vi "Periodic Tasks.vi"(8 "error in":errorcluster) -> ()   [LabVIEW 2020]
doc: "This VI runs in parallel to other tasks. It can contain as many user-defined periodic loops as you need. These can carry out PID or other sorts of timed response."
uses:
  <vilib>/Rock Robotics/WPI/Utilities/WPI_GetSetVariantRefNum.vi
  <vilib>/Rock Robotics/WPI/ThirdParty/REV Robotics/REVLib/Typedef/Spark MAX Control Type.ctl
  981LabViewComponents/2022 Robot Global Data.vi
panel:
  out "Sensor Position":dbl
  out "Sensor Velocity":dbl
  out "YRPHfH":T1
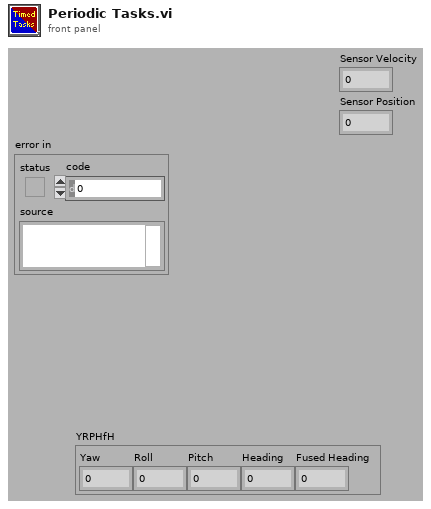
[diagram p1: front panel]
types:
  T1 = cluster{"Yaw":dbl, "Roll":dbl, "Pitch":dbl, "Heading":dbl, "Fused Heading":dbl}
  T2 = typedef "WPI_MotorControlDeviceRef.ctl" = cluster{"DeviceStatus":errorcluster, "Type":T3, "PWM":cluster{"PWM Channel":T4, "DeadBand":T5}, "CAN":cluster{"Device Number":u8, "SetOutput VI Ref":variant, "GetOutput VI Ref":variant, "Enable VI Ref":variant, "Disable VI Ref":variant, "Data":variant}, "Invert":bool, "DIO PWM":cluster{"PWM \"Enable\" Channel":T4, "DIOChannel":T6, "PWM Rate":dbl}}
  T3 = typedef "WPI_MotorControlType.ctl" = enum16{"PWM", "CAN", "DIO PWM"}
  T4 = typedef "FPGA_DIOPWMChannel.ctl" = enum8{"PWM 0", "PWM 1", "PWM 2", "PWM 3", "PWM 4", "PWM 5", "PWM 6", "PWM 7", "PWM 8", "PWM 9", "PWM MXP 0", "PWM MXP 1", "PWM MXP 2", "PWM MXP 3", "PWM MXP 4", "PWM MXP 5", "PWM MXP 6", "PWM MXP 7", "PWM MXP 8", "PWM MXP 9", "Invalid"}
  T5 = typedef "WPI_PWMDeadband.ctl" = cluster{"Name":string, "maxPositivePwm":i32, "minPositivePwm":i32, "centerPwm":i32, "maxNegativePwm":i32, "minNegativePwm":i32, "angularRange":u16}
  T6 = typedef "FPGA_DIOChannel.ctl" = enum8{"DIO 0", "DIO 1", "DIO 2", "DIO 3", "DIO 4", "DIO 5", "DIO 6", "DIO 7", "DIO 8", "DIO 9", "DIO MXP 0", "DIO MXP 1", "DIO MXP 2", "DIO MXP 3", "DIO MXP 4", "DIO MXP 5", "DIO MXP 6", "DIO MXP 7", "DIO MXP 8", "DIO MXP 9", "DIO MXP 10", "DIO MXP 11", "DIO MXP 12", "DIO MXP 13", "DIO MXP 14", "DIO MXP 15", "SPI Port CS1", "SPI Port CS2", "SPI Port CS3", "SPI Port MISO", "SPI Port MOSI", "Invalid"}
  T7 = typedef "WPI_JoystickDevRef.ctl" = cluster{"Device":T8}
  T8 = typedef "WPI_JoystickDeviceEnum.ctl" = enum16{"USB 0", "USB 1", "USB 2", "USB 3", "USB 4", "USB 5"}
  T9 = cluster{"JoystickDevRef":T7, "MotorControlDevRef":T2}
  T10 = cluster{"P Gain":dbl, "I Gain":dbl, "D Gain":dbl, "F Gain":dbl, "I Zone":dbl, "Min Output":dbl, "Max Output":dbl}
  T11 = typedef "Spark MAX Control Type.ctl" = enum16{"Percent VBus", "Voltage", "Velocity", "Position", "Smart Motion", "Current", "Smart Velocity"}
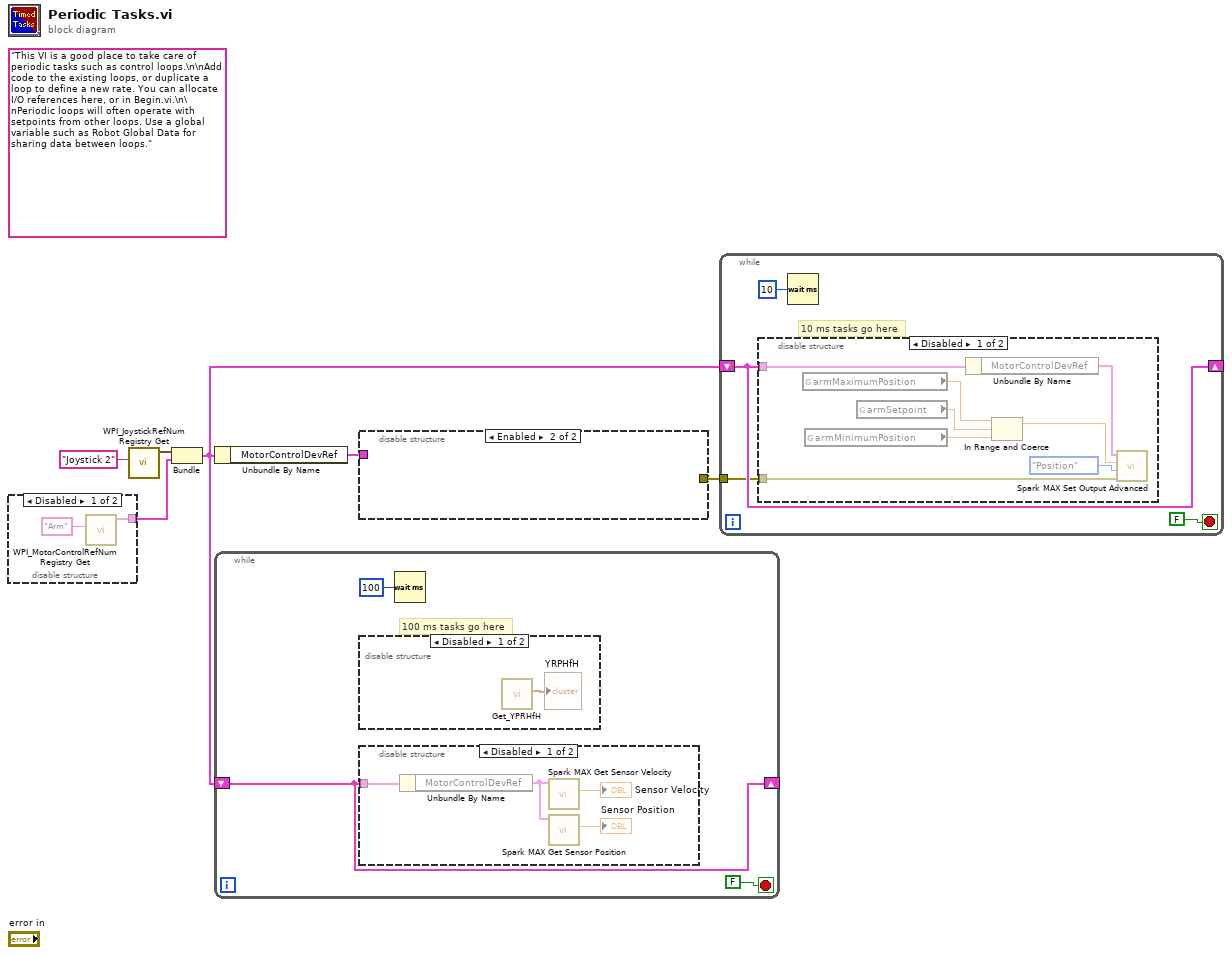
[diagram p0: block diagram]
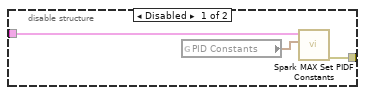
[diagram p3: hidden frame]
diagram:
  (unwired) "This VI is a good place to take care of periodic tasks such as control loops.\n\nAdd code to the existing loops, or duplicate a loop to define a new rate. You can allocate I/O references here, or in Begin.vi.\n\nPeriodic loops will often operate with setpoints from other loops. Use a global variable such as Robot Global Data for sharing data between loops."
  n1 = disable-structure shown="Disabled" {
    disable-tunnel: [w8 _] -> w4
    frame Disabled {
      n2 = call <vilib>:"WPI_MotorControlRefNum Registry Get.vi"("refnum name"="Arm") -> ("MotorControlDevRef"=w8:T2)  [unwired: 9 in, 1 out]
    }
    frame Enabled {
    }
  }
  n3 = call <vilib>:"WPI_JoystickRefNum Registry Get.vi"("refnum name"="Joystick 2") -> ("JoystickDevRef"=w5:T7)  [unwired: 1 in, 9 out]
  n4 = Bundle("JoystickDevRef"=w5, "MotorControlDevRef"=w4) -> (w3:T9)  [unwired: 1 out]
  n5 = Unbundle By Name(w3) -> ("MotorControlDevRef"=w2:T2)
  n6 = while {
    shift-right: [w9] -> _
    shift-left: w3 -> [w9]
    stop <- FALSE stop-if-true
    # "100 ms tasks go here"
    n7 = disable-structure shown="Disabled" {
      frame Disabled {
        n8 = call <vilib>:"Get_YPRHfH.vi"() -> ("YRPHfH"=→"YRPHfH":T1)  [unwired: 11 in]
      }
      frame Enabled {
      }
    }
    n9 = disable-structure shown="Disabled" {
      disable-tunnel: w9 -> [w13 _]
      frame Disabled {
        n10 = Unbundle By Name(w13) -> ("MotorControlDevRef"=w12:T2)
        n11 = call <vilib>:"Spark MAX Get Sensor Velocity.vi"("MotorControlDevRef in"=w12) -> ("Sensor Velocity"=→"Sensor Velocity":dbl)  [unwired: 7 in, 3 out]
        n12 = call <vilib>:"Spark MAX Get Sensor Position.vi"("MotorControlDevRef in"=w12) -> ("Sensor Position"=→"Sensor Position":dbl)  [unwired: 7 in, 3 out]
      }
      frame Enabled {
      }
    }
    n13 = Wait (ms)(milliseconds to wait=u32 100) -> ()  [unwired: 1 out]
  }
  n14 = disable-structure shown="Enabled" {
    disable-tunnel: w2 -> [w18 _]
    disable-tunnel: [w17 _] -> w1
    frame Disabled {
      n15 = global read "2022 Robot Global Data.vi" "PID Constants"() -> (w19:T10)
      n16 = call <vilib>:"Spark MAX Set PIDF Constants.vi"("PID Constants"=w19, "MotorControlDeviceRef"=w18) -> ("error out"=w17:errorcluster)  [unwired: 8 in, 1 out]
    }
    frame Enabled {
    }
  }
  n17 = while {
    shift-right: [w21] -> _
    shift-left: w3 -> [w21]
    tunnel: w1 -> [w20]
    stop <- FALSE stop-if-true
    # "10 ms tasks go here"
    n18 = disable-structure shown="Disabled" {
      disable-tunnel: w21 -> [w30 _]
      disable-tunnel: w20 -> [w24 _]
      frame Disabled {
        n19 = global read "2022 Robot Global Data.vi" "armMaximumPosition"() -> (w29:dbl)
        n20 = global read "2022 Robot Global Data.vi" "armMinimumPosition"() -> (w28:dbl)
        n21 = global read "2022 Robot Global Data.vi" "armSetpoint"() -> (w27:dbl)
        n22 = Unbundle By Name(w30) -> ("MotorControlDevRef"=w25:T2)
        n23 = In Range and Coerce(upper limit=w29, x=w27, lower limit=w28) -> (coerced(x)=w26:dbl)  [unwired: 1 out]
        n24 = call <vilib>:"Spark MAX Set Output Advanced.vi"("error in (no error)"=w24, "Control Mode"=Spark_MAX_Control_Type."Position", "Setpoint"=w26, "MotorControlDevRef"=w25) -> ()  [unwired: 6 in, 2 out]
      }
      frame Enabled {
      }
    }
    n25 = Wait (ms)(milliseconds to wait=u32 10) -> ()  [unwired: 1 out]
  }
